vi "LinkamStageController.vi"() -> ()   [LabVIEW 2013]
doc: "The Grab and Save to AVI VI acquires images continuously using the high-level acquisition VIs, displays them in an image control, and saves the images to an AVI file. A grab is appropriate for high-speed applications that process only one image at a time. Use an AVI file to save multiple images to a single file for post-processing or record images.\n\nIMAQ Init initializes the device. IMAQ Grab Setup initializes the grab function and starts capturing images to an internal software buffer. IMAQ Create creates an image buffer IMAQ Grab Acquire copies the internal buffer to Image out, and an image control displays the image on the front panel. IMAQ Close releases resources associated with the acquisition, and IMAQ Dispose frees the image buffer.\n\nIMAQ AVI Create initializes the AVI file, IMAQ AVI WriteFrame adds each image to the AVI file, and IMAQ AVI Close completes writing to the AVI file. Call IMAQ AVI Create for each AVI file created."
uses:
  <vilib>/userdefined/High Color/IMAQdx.ctl
  Mag.ctl
  <vilib>/Instr/_visa.llb/VISA Open Access Mode.ctl
  ImageEnum4GFV.ctl
  RampProgramModel/RampProgramModel.lvclass
  AVI recoder state.ctl
  <vilib>/vision/Avi.llb/IMAQ AVI2 Refnum.ctl
  DateandTime.ctl
  RampProgramModel/RampProgramModel.lvclass/RampProgramModel.ctl
  TextOnImage.ctl
  Ascii Experiment Data.ctl
  RampState.ctl
  <vilib>/Instr/_visa.llb/VISA Configure Serial Port (Instr).vi
  <vilib>/Utility/file.llb/Read From Spreadsheet File (DBL).vi
  <vilib>/Utility/file.llb/Write To Spreadsheet File (string).vi
  <vilib>/vision/driver/NI_Vision_Acquisition_Software.lvlib
  <resource>/objmgr/imaqdx.rc
panel:
  in  "Stop Recording\n@ Temp (°C)":dbl=5.0 format="%#_g °C"
  in  "Start Recording\n@ Temp (°C)":dbl=-2.0 format="%#_g °C"
  in  "Enable\nAutomatic\nRecording":bool=TRUE
  in  "Gain (0-570)":dbl=300.0 min=0.0 max=570.0 step=1.0
  in  "Shutter (1-4095)":dbl=4095.0 min=1.0 max=4095.0 step=1.0
  in  "High Resolution":bool
  in  "Remarks":string
  out "Goal":string
  out "Experiment Name":string
  in  "NewExperiment":bool
  out "File Path":path=path "E:/LINKAM Measurements_Naama"
  in  "Mag":T1=enum."20x_LM"
  out "Temp Chart":dbl(graph)
  out "Time Remaining\n(HH:MM:SS)":dbl format="%<%H:%M:%S>t"
  out "Ramp Program Table":string[][](table)
  in  "Clear Table":bool
  in  "Add Entry":bool
  in  "StopProgram":bool
  in  "RunProgram":bool
  in  "PauseProgram":bool
  in  "SaveProgram":bool
  in  "LoadProgram":bool
  in  "Cycles":u32=1 min=1 max=1000 step=1
  out "Cycle No.":u32 min=1 max=1000 step=1
  in  "Pump Speed":u8(slide) max=30 step=1 scale=0.0..30.0
  in  "DelayInComm(ms)":u32=50
  out "Video Grabber":bool
  out "Linkam Controller":bool
  out "Ramp Controller":bool
  out "Video Recorder":bool
  in  "Pause":bool caption="Start Cooling/Heating"
  in  "Stop":bool caption="Start Cooling/Heating"
  in  "Record":bool caption="Start Cooling/Heating"
  out "Status":string="Stop"
  in  "TakeRefImage":bool caption="Start Cooling/Heating"
  in  "Time Between Consecutive Frames (sec)":dbl=1.0 caption="Time Between \nConsecutive \nFrames (sec)" min=0.0 max=3600.0 step=0.01 format="%.2g s"
  out "Full avi Path and Name":path=path "Z:/Downloads/data/Test-18_05_2014-15_02_54.avi"
  out "Codec Type":string="Motion JPEG (NI Vision)"
  in  "index 2":i32=4
  in  "error in (no error) 2":errorcluster
  out "Status":string="Stopped"
  out "Repeat Program ind":u32=1 min=1 max=1000 step=1
  in  "error in (no error)":errorcluster
  out "Reference Image":T2(plugin-control)
  in  "Hold Cooling/Heating":bool caption="Start Cooling/Heating"
  in  "Stop Cooling/Heating":bool caption="Start Cooling/Heating"
  in  "Start Cooling/Heating":bool
  in  "Setpoint (°C)":dbl=28.0 min=-50.0 max=50.0 step=0.1 format="%.1g °C"
  in  "Cooling Rate (°C/min)":dbl=1.0 min=0.0 max=20.0 step=0.01 format="%.2g °C/min"
  out "Current Temp (°C)":dbl=27.0 format="%.1g °C"
  out "Status of Liquied Nitrogen Pump":string="33"
  in  "Max Speed":bool
  in  "LNP mode":bool=TRUE
  out "Error Message":string
  out "Status of Temperature Controller":string="Setpoint"
  out "Temp String (C)":string="27.0"
  out "Timer":u32=9
  out "remaining string":string="010E"
  out "read buffer":string="0€Á€€€010E\r"
  out "return count":u32=11
  in  "Session In":T3="cam0"
  out "Image":T2(plugin-control)
  in  "stop":bool
  # "Live Image"
  # "Reference Image"
  # "Select your Camera above"
  # "Linkam Temperature Controller"
  # "Experiment Data"
  # "Video Recorder"
  # "Engines Status"
  # "Status"
  # "Liquid Nitrogen Pump Controller"
  # "Pump Speed"
  # "Video Grabber"
  # "Error Message"
  # "Ramp Table Controller"
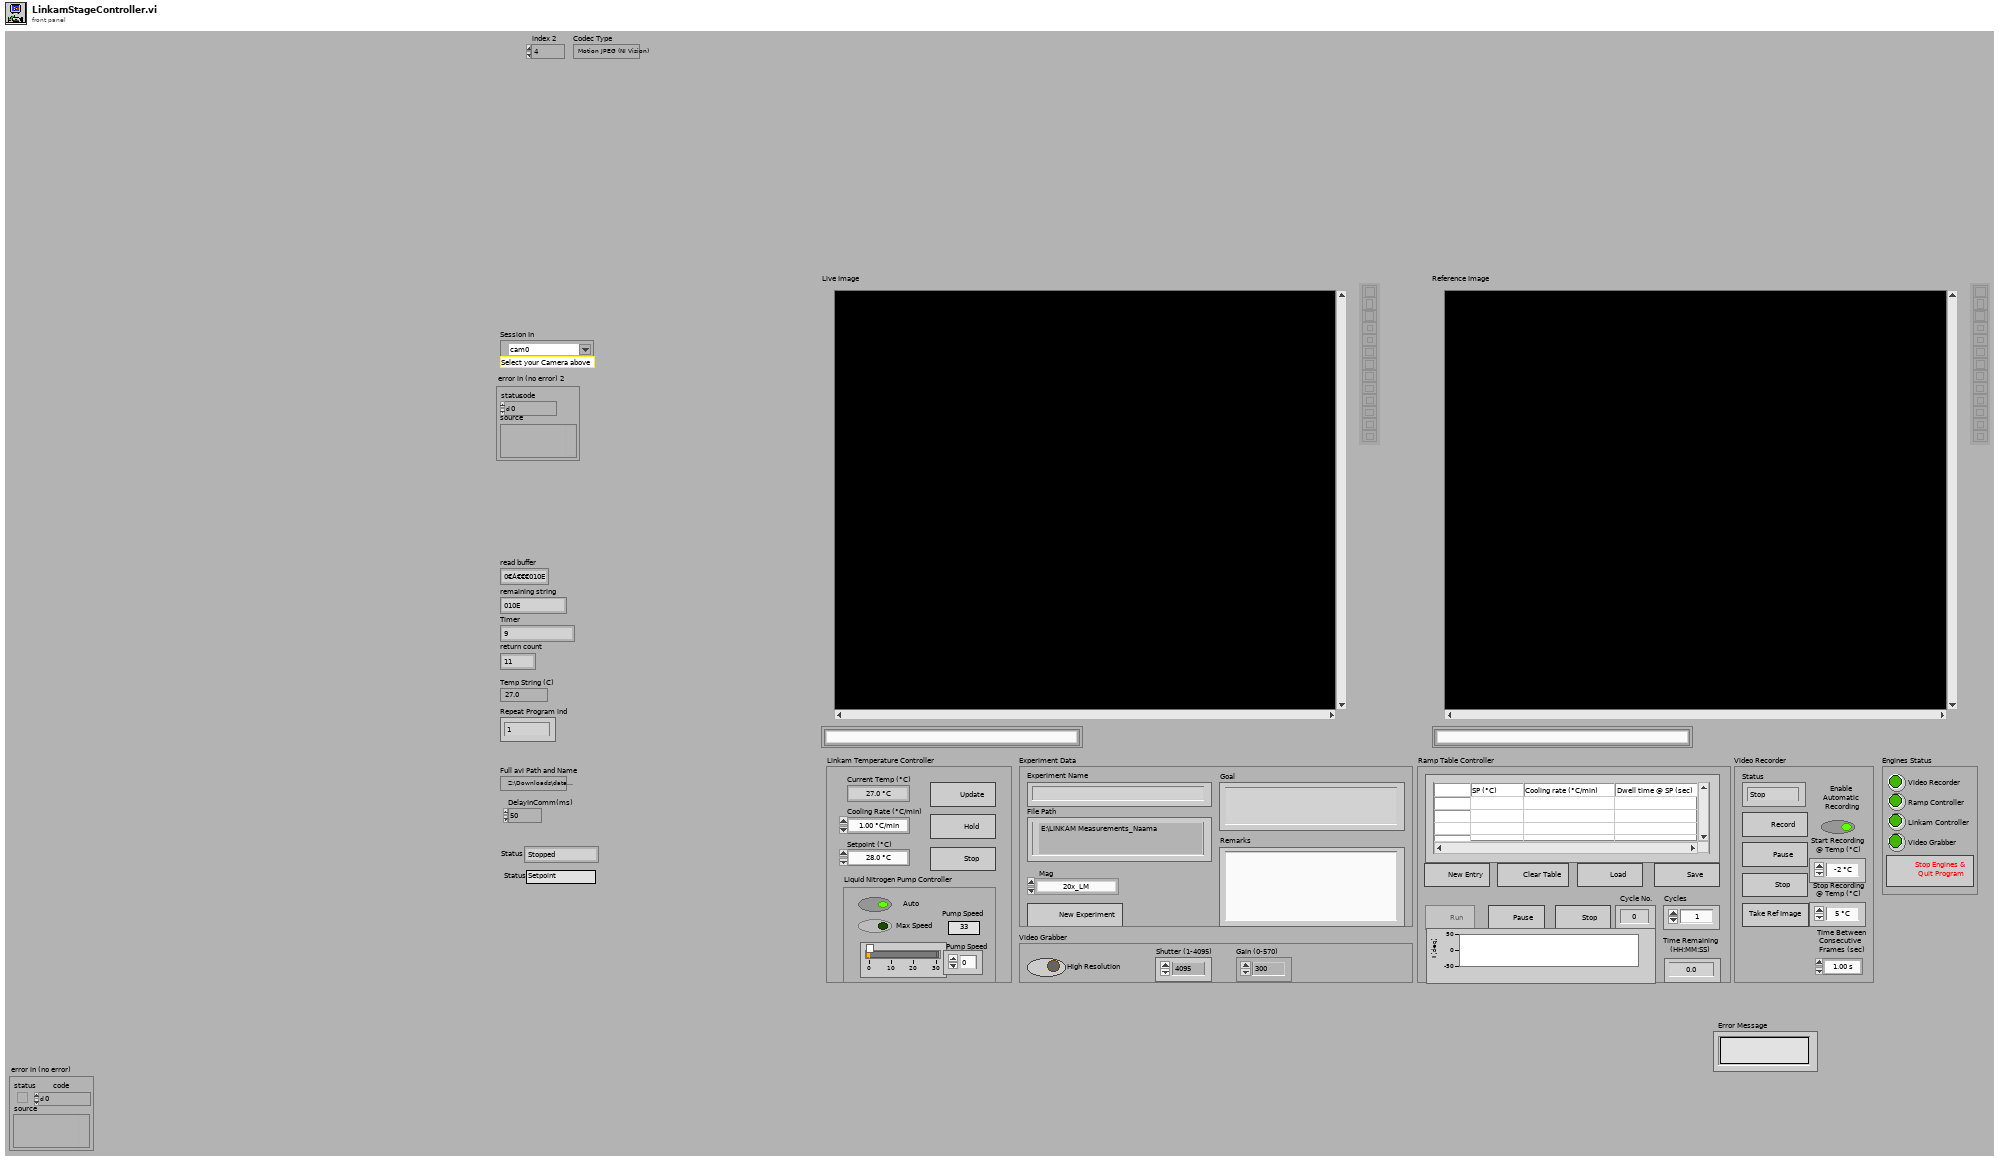
[diagram p1: front panel]
types:
  T1 = typedef "Mag.ctl" = enum16{"5x_M_BD", "10x_M", "10xM_BD", "10x_ph1", "20x_S", "20x_LM", "50x_S"}
  T2 = typedef "IMAQ Image.ctl" = refnum<image>
  T3 = typedef "IMAQdx.ctl" = refnum<k21>
  T4 = enum8{"Enabled", "Disabled", "Disabled and Grayed Out"}
  T5 = typedef "DateandTime.ctl" = cluster{"Date and Time":string, "Temp (deg)":string}[]
  T6 = typedef "IMAQ AVI2 Refnum.ctl" = refnum<k20>
  T7 = typedef "AVI recoder state.ctl" = enum16{"Record", "Pause", "Stop", "Init"}
  T8 = typedef "ImageEnum4GFV.ctl" = enum16{"Delete", "Write", "Read", "Init"}
  T9 = typedef "VISA Open Access Mode.ctl" = u32
  T10 = typedef "RampState.ctl" = enum16{"Pause Program", "Heatling/Cooling", "Dwelling @ SP", "Stopped"}
  T11 = typedef "Ascii Experiment Data.ctl" = cluster{"Experiment Name":string, "Goal":string, "Remarks":string, "File Path":string, "Mag":string, "Repeat Program Number":string, "Full avi Path and Name":path, "Ramp Table ":string[][], "Date and Time":T5}
  T12 = cluster{"date/time string":string, "Temp String (C)":string}
  T13 = typedef "TextOnImage.ctl" = cluster{"Status":string, "Experiment Name":string, "Current Temp (C)":string, "Set Point (C)":string, "Cooling Rate (C/min)":string, "Mag":T1}
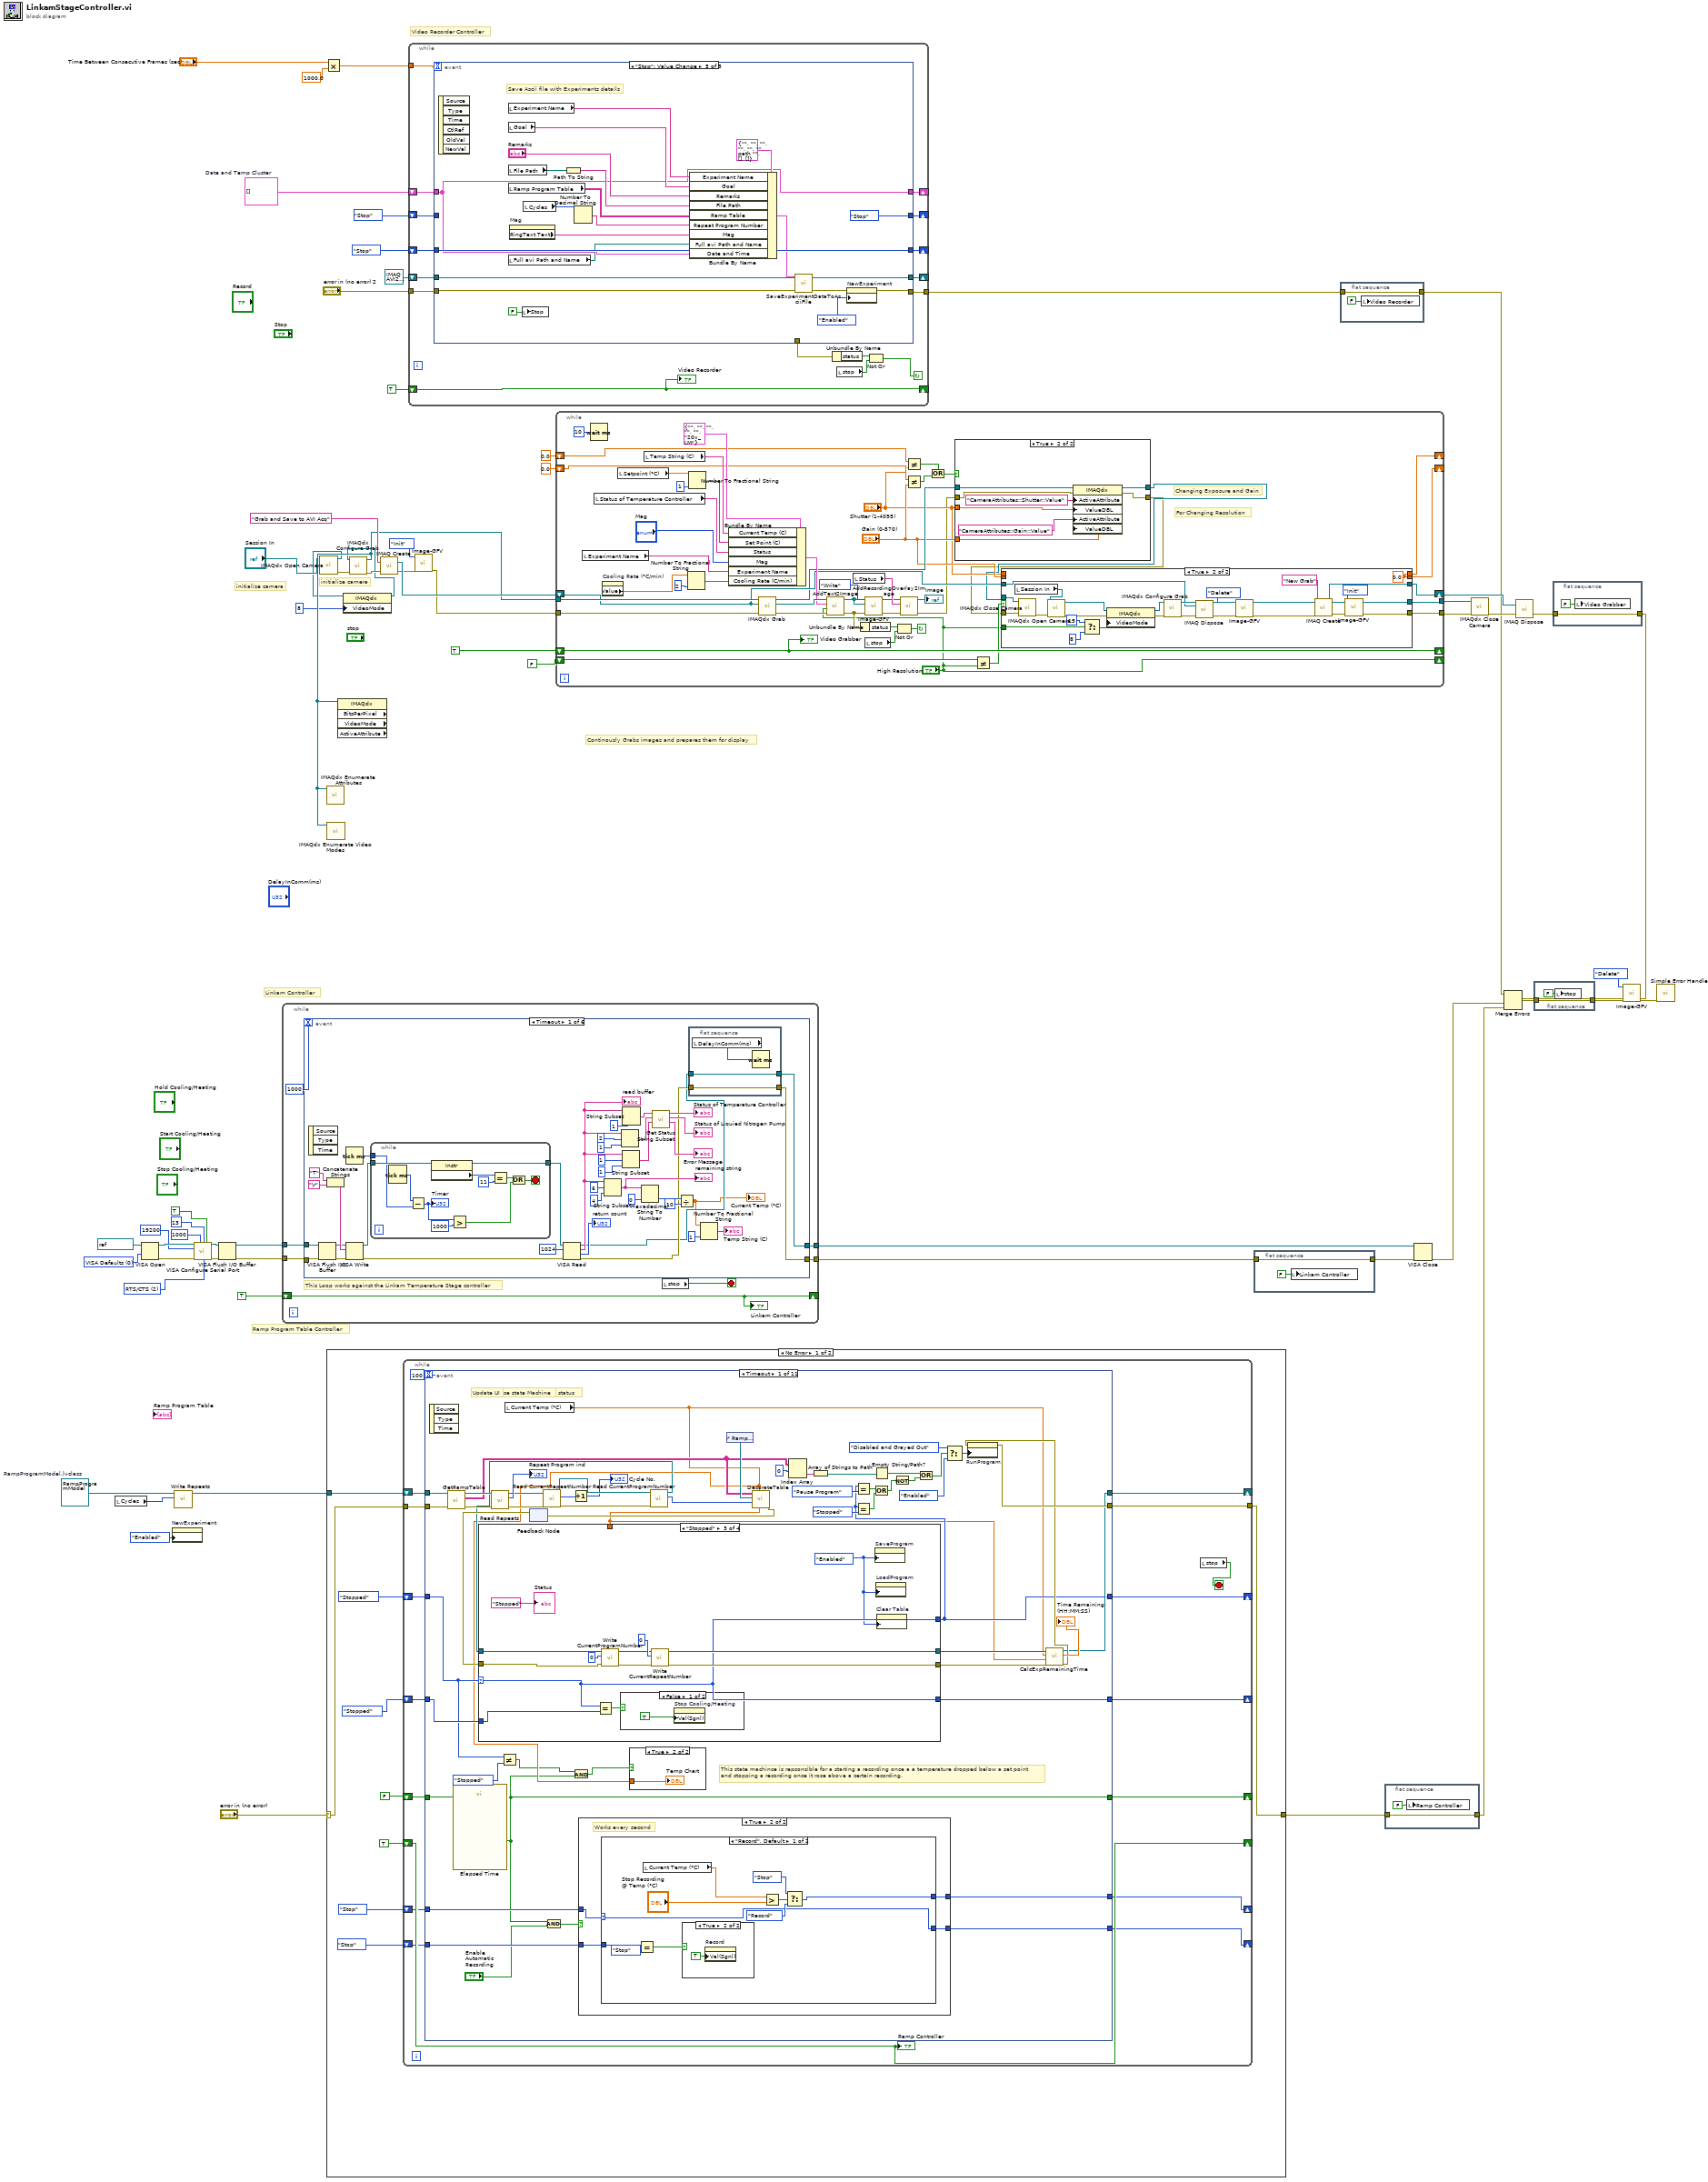
[diagram p0: block diagram]
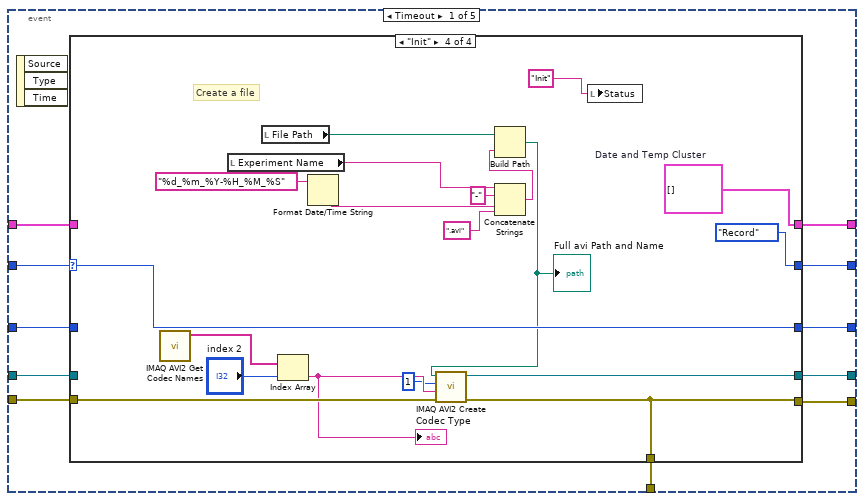
[diagram p2: hidden frame]
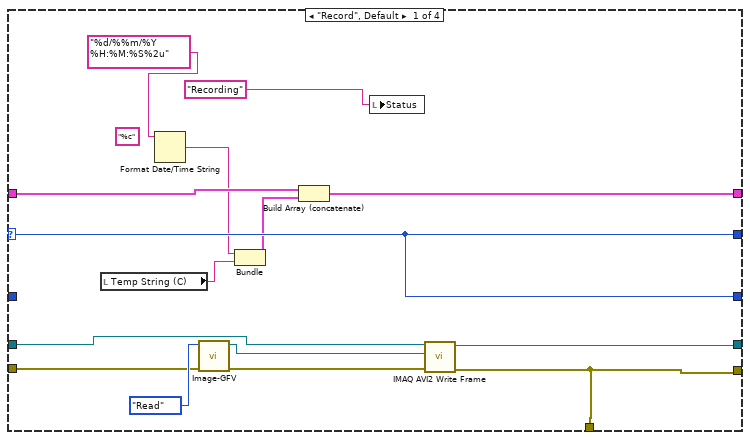
[diagram p3: hidden frame]
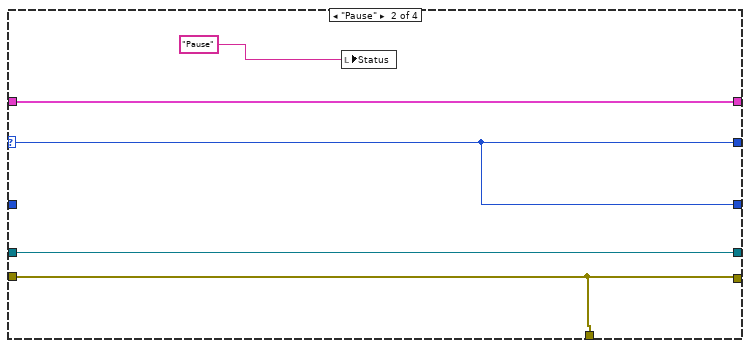
[diagram p4: hidden frame]
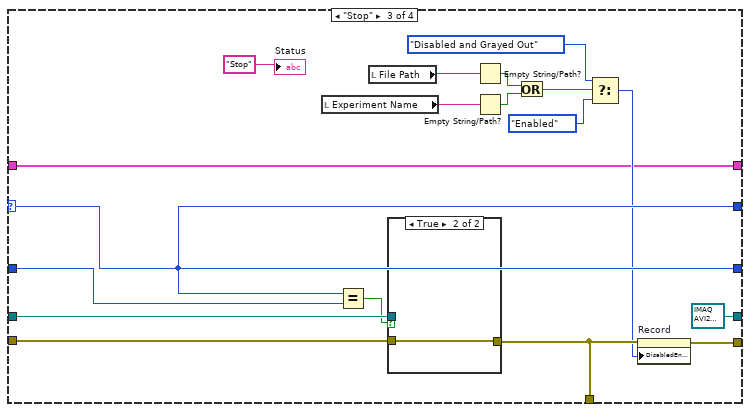
[diagram p5: hidden frame]
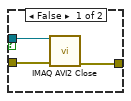
[diagram p6: hidden frame]
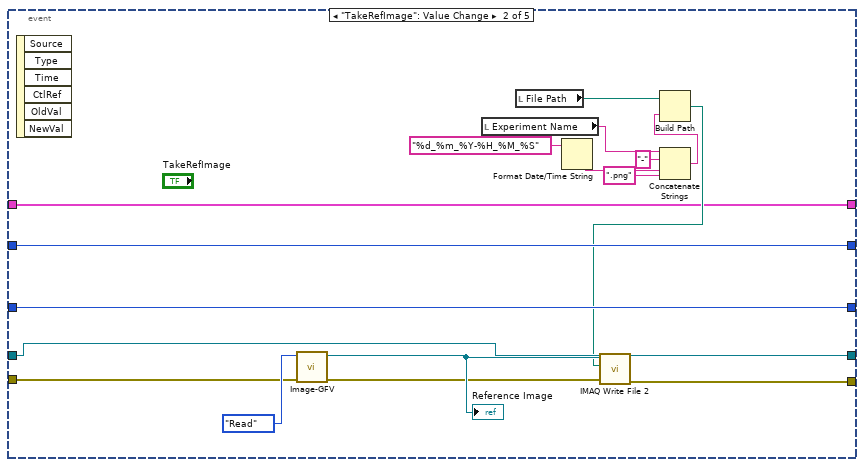
[diagram p7: hidden frame]
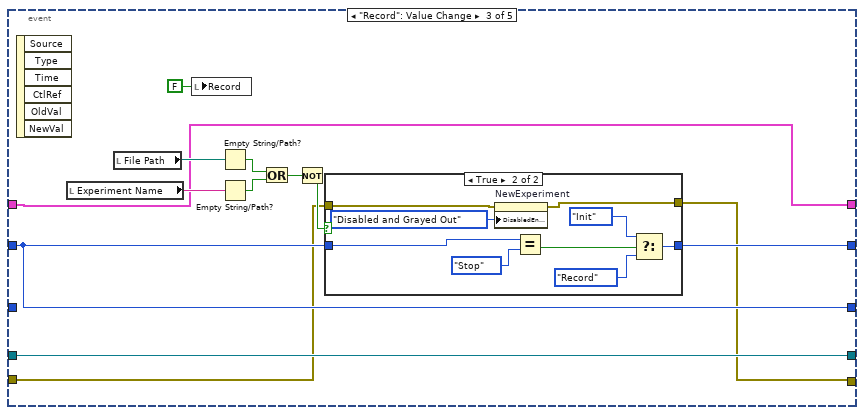
[diagram p8: hidden frame]
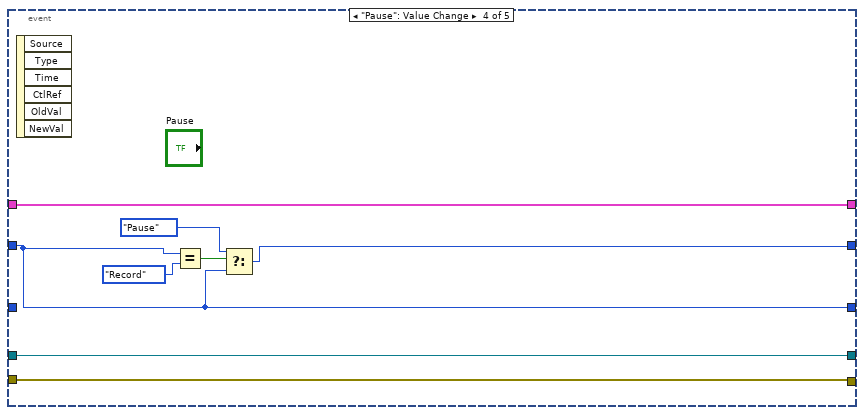
[diagram p10: hidden frame]
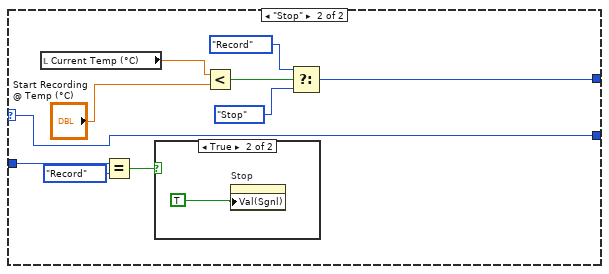
[diagram p13: hidden frame]
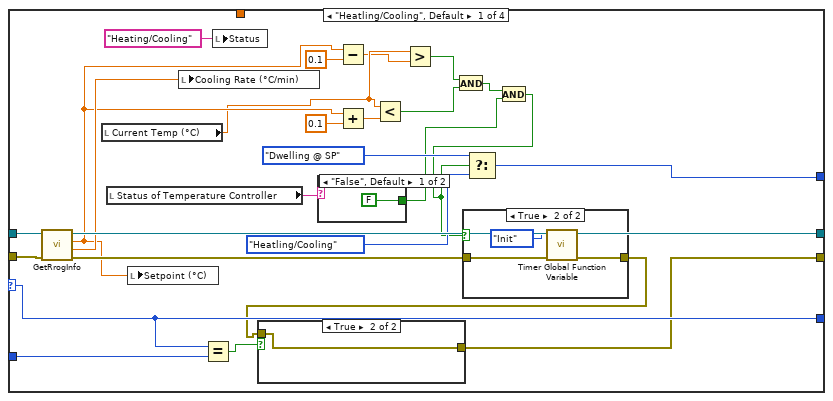
[diagram p16: hidden frame]
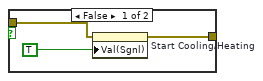
[diagram p17: hidden frame]
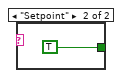
[diagram p18: hidden frame]
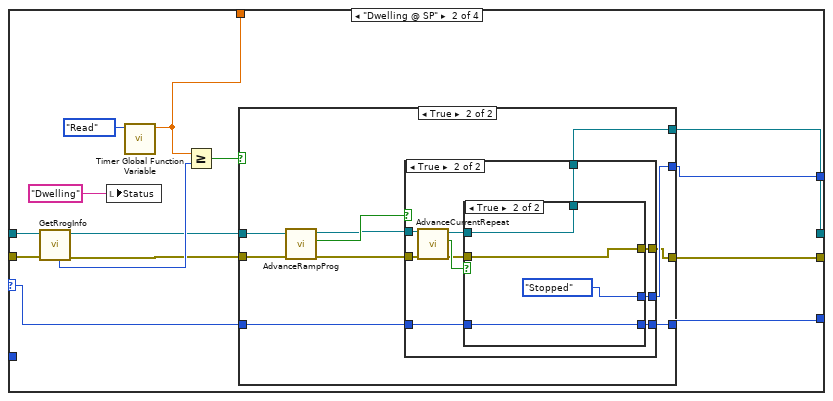
[diagram p20: hidden frame]
diagram:
  w11 = T5 []  # Date and Temp Cluster
  w33 = refnum<class "RampProgramModel.lvclass"> refnum  # RampProgramModel.lvclass
  w53 = T9 0 items=["VISA Defaults"=0, "Exclusive Lock"=1, "Load Configured Settings"=4] ("Access Mode")
  w57 = u16 2 items=["None", "XON/XOFF", "RTS/CTS", "XON/XOFF & RTS/CTS", "DTR/DSR", "XON/XOFF & DTR/DSR"] ("flow control (0:none)")
  # "Linkam Controller"
  # "Video Recorder Controller"
  # "Ramp Program Table Controller"
  # "Continously Grabs images and prepares them for display"
  # "initialize camera"
  # "initialize camera"
  n1 = local read "Cycles"() -> (w34:u32)
  n2 = VISA Open(access mode=w53, VISA resource name=refnum<visa-resource-name> "COM1") -> (VISA resource name=w60:refnum<visa-resource-name>, error out=w61:errorcluster)  [unwired: 3 in]
  n3 = property on="NewExperiment" class="Bool"("DisabledEnum"=T4."Enabled" ("Disabled")) -> ()  [unwired: 2 in, 2 out]
  n4 = call "Write Repeats.vi"("Repeats"=w34, "RampProgramModel in"=w33) -> ("RampProgramModel out"=w32:refnum<class "RampProgramModel.lvclass">)  [unwired: 8 in, 1 out]
  n5 = call-poly "VISA Configure Serial Port"("VISA resource name"=w60, "timeout (10sec)"=u32 1000, "termination char\n(0xA = '\\n' = LF)"=u8 13 ("termination char\n(0xA = '\\n' = LF)"), "Enable Termination\nChar (T)"=TRUE ("Enable Termination\nChar (T)"), "baud rate (9600)"=u32 19200, "error in (no error)"=w61, "flow control (0:none)"=w57) -> ("VISA resource name out"=w52:refnum<visa-resource-name>, "error out"=w51:errorcluster)  [unwired: 7 in]
  n6 = VISA Flush I/O Buffer(VISA resource name=w52, error in (no error)=w51) -> (VISA resource name out=w50:refnum<visa-resource-name>, error out=w49:errorcluster)  [unwired: 1 in]
  n7 = while {
    tunnel: [w69] -> w55
    tunnel: [w68] -> w17
    tunnel: w50 -> [w67]
    tunnel: w49 -> [w66]
    shift-right: [w63] -> _
    shift-left: TRUE -> [w63]
    stop <- w65 stop-if-true
    # "This Loop works against the Linkam Temperature Stage controller"
    n8 = event shown="[0] Timeout" {
      selector: _ -> [_ _ _ _ _ _]
      dyn-events: _ -> [_ _ _ _ _ _]
      timeout: 1000 -> [_ _ _ _ _ _]
      tunnel: [w72 w123 w136 w160 w182 w186] -> w69
      tunnel: [w71 w122 w135 w159 w183 w185] -> w68
      tunnel: w67 -> [w92 w131 w144 w171 w182 w210]
      tunnel: w66 -> [w91 w130 w143 w170 w183 w209]
      event Timeout {
        n9 = event-data() -> ()  [unwired: 1 in, 3 out]
        n10 = VISA Flush I/O Buffer(VISA resource name=w92, error in (no error)=w91) -> (VISA resource name out=w90:refnum<visa-resource-name>, error out=w89:errorcluster)  [unwired: 1 in]
        n11 = Concatenate Strings("T" ("write buffer"), "\r") -> (w93:string)
        n12 = Tick Count (ms)() -> (millisecond timer value=w96:u32)
        n13 = VISA Write(VISA resource name=w90, write buffer=w93, error in (no error)=w89) -> (VISA resource name out=w99:refnum<visa-resource-name>, error out=w97:errorcluster)  [unwired: 1 out]
        n14 = while {
          tunnel: w99 -> [w114]
          tunnel: [w113] -> w98
          tunnel: w96 -> [w112]
          stop <- w115 stop-if-true
          n15 = Tick Count (ms)() -> (millisecond timer value=w119:u32)
          n16 = Subtract(x=w119, y=w112) -> (x-y=w111:u32)
          "Timer" <- w111
          n17 = property class="Instr"(reference=w114) -> (reference out=w113:refnum<visa-resource-name>, "Serial Settings:Number of Bytes at Serial Port"=w121:u32)  [unwired: 1 in, 1 out]
          n18 = Greater?(x=w111, y=u32 1000) -> (0:w116:bool)
          n19 = Equal?(x=w121, y=u32 11) -> (x = y?=w117:bool)
          n20 = Or(x=w117, y=w116) -> (x .or. y?=w115:bool)
        }
        n21 = VISA Read(VISA resource name=w98, byte count=u32 1024, error in (no error)=w97) -> (VISA resource name out=w73:refnum<visa-resource-name>, read buffer=w77:string, return count=→"return count":u32, error out=w74:errorcluster)
        "read buffer" <- w77
        n22 = String Subset(string=w77, offset (0)=6, length (rest)=4 ("length (rest)")) -> (substring=w102:string)
        "remaining string" <- w102
        n23 = String Subset(string=w77, offset (0)=2, length (rest)=1 ("length (rest)")) -> (substring=w81:string)
        n24 = String Subset(string=w77, offset (0)=1, length (rest)=1 ("length (rest)")) -> (substring=w76:string)
        n25 = String Subset(string=w77, length (rest)=1 ("length (rest)")) -> (substring=w85:string)  [unwired: 1 in]
        n26 = Hexadecimal String To Number(string=w102, default (0uL)=i16 0 ("default (0 U32)")) -> (number=w101:i16)  [unwired: 1 in, 1 out]
        n27 = call "Get Status.vi"("Error message input"=w76, "Input Pump Status string"=w81, "Input Status String"=w85) -> ("Error message string"=→"Error Message":string, "Output Pump Status"=→"Status of Liquied Nitrogen Pump":string, "Output Status String"=→"Status of Temperature Controller":string)  [unwired: 6 in]
        n28 = Divide(x=w101, y=i16 10) -> (x/y=w70:dbl)
        "Current Temp (°C)" <- w70
        n29 = flat-sequence {
          tunnel: w74 -> [w110]
          tunnel: [w110] -> w71
          tunnel: w73 -> [w109]
          tunnel: [w109] -> w72
          frame #0 {
            n30 = local read "DelayInComm(ms)"() -> (w108:u32)
            n31 = Wait (ms)(milliseconds to wait=w108) -> ()  [unwired: 1 out]
          }
        }
        n32 = Number To Fractional String(number=w70, precision (6)=i16 1) -> (F-format string=→"Temp String (C)":string)  [unwired: 2 in]
      }
      event "Stop Cooling/Heating": Value Change {
        n33 = event-data() -> ()  [unwired: 1 in, 6 out]
        n34 = Concatenate Strings("E" ("write buffer"), "\r") -> (w127:string)
        n35 = VISA Write(VISA resource name=w131, write buffer=w127, error in (no error)=w130) -> (VISA resource name out=w125:refnum<visa-resource-name>, error out=w124:errorcluster)  [unwired: 1 out]
        n36 = flat-sequence {
          tunnel: w124 -> [w134]
          tunnel: [w134] -> w122
          tunnel: w125 -> [w133]
          tunnel: [w133] -> w123
          frame #0 {
            n37 = local read "DelayInComm(ms)"() -> (w132:u32)
            n38 = Wait (ms)(milliseconds to wait=w132) -> ()  [unwired: 1 out]
          }
        }
        n39 = local write "Stop Cooling/Heating"(FALSE ("Stop Cooling/Heating")) -> ()
      }
      event "Hold Cooling/Heating": Value Change {
        n40 = event-data() -> ()  [unwired: 1 in, 6 out]
        n41 = Concatenate Strings("OCR" ("write buffer"), "\r") -> (w140:string)
        n42 = VISA Write(VISA resource name=w144, write buffer=w140, error in (no error)=w143) -> (VISA resource name out=w138:refnum<visa-resource-name>, error out=w137:errorcluster)  [unwired: 1 out]
        n43 = local write "Hold Cooling/Heating"(FALSE ("Hold Cooling/Heating")) -> ()
        n44 = flat-sequence {
          tunnel: w137 -> [w147]
          tunnel: [w147] -> w135
          tunnel: w138 -> [w146]
          tunnel: [w146] -> w136
          frame #0 {
            n45 = local read "DelayInComm(ms)"() -> (w145:u32)
            n46 = Wait (ms)(milliseconds to wait=w145) -> ()  [unwired: 1 out]
          }
        }
      }
      event "LNP mode", "Pump Speed": Value Change {
        n47 = event-data() -> ()  [unwired: 1 in, 6 out]
        n48 = Select(t="Pa0", s="LNP mode", f="Pm0") -> (s? t:f=w166:string)
        n49 = Concatenate Strings(w166, "\r") -> (w168:string)
        n50 = VISA Write(VISA resource name=w171, write buffer=w168, error in (no error)=w170) -> (VISA resource name out=w158:refnum<visa-resource-name>, error out=w157:errorcluster)  [unwired: 1 out]
        n51 = flat-sequence {
          tunnel: w157 -> [w174]
          tunnel: [w174] -> w156
          tunnel: w158 -> [w173]
          tunnel: [w173] -> w155
          frame #0 {
            n52 = local read "DelayInComm(ms)"() -> (w172:u32)
            n53 = Wait (ms)(milliseconds to wait=w172) -> ()  [unwired: 1 out]
          }
        }
        n54 = Add(x="Pump Speed", y=u8 48) -> (x+y=w152:u8)
        n55 = Type Cast(x=w152) -> (*(type *) &x=w150:string)  [unwired: 1 out]
        n56 = Concatenate Strings("P" ("string"), w150) -> (w149:string)
        n57 = Concatenate Strings(w149, "\r") -> (w163:string)
        n58 = VISA Write(VISA resource name=w155, write buffer=w163, error in (no error)=w156) -> (VISA resource name out=w162:refnum<visa-resource-name>, error out=w161:errorcluster)  [unwired: 1 out]
        n59 = flat-sequence {
          tunnel: w161 -> [w177]
          tunnel: [w177] -> w159
          tunnel: w162 -> [w176]
          tunnel: [w176] -> w160
          frame #0 {
            n60 = local read "DelayInComm(ms)"() -> (w175:u32)
            n61 = Wait (ms)(milliseconds to wait=w175) -> ()  [unwired: 1 out]
          }
        }
      }
      event "Max Speed": Value Change {
        n62 = event-data() -> ()  [unwired: 1 in, 6 out]
        n63 = Select(t=u8 30 ("f"), s="Max Speed", f=u8 0) -> (s? t:f=w180:u8)
        n64 = property on="Pump Speed" class="Slide (strict)"("Val(Sgnl)"=w180) -> ()  [unwired: 2 in, 2 out]
      }
      event "Start Cooling/Heating": Value Change {
        # "Caused to max speed at every update"
        n65 = event-data() -> ()  [unwired: 1 in, 6 out]
        n66 = Multiply(x="Cooling Rate (°C/min)", y=u16 100) -> (x*y=w199:dbl)
        n67 = To Long Integer(number=w199) -> (32bit integer=w198:i32)
        n68 = Number To Decimal String(number=w198) -> (decimal integer string=w211:string)  [unwired: 1 in]
        n69 = property on="LNP mode" class="Bool (strict)"() -> ("Value"=w184:bool)  [unwired: 2 in, 2 out]
        n70 = Concatenate Strings("R1" ("write buffer"), w211, "\r") -> (w208:string)
        n71 = VISA Write(VISA resource name=w210, write buffer=w208, error in (no error)=w209) -> (VISA resource name out=w195:refnum<visa-resource-name>, error out=w196:errorcluster)  [unwired: 1 out]
        n72 = case shown="False" w184 {
          frame False {
            n73 = property on="LNP mode" class="Bool (strict)"("Val(Sgnl)"=TRUE ("LNP mode")) -> ()  [unwired: 2 in, 2 out]
          }
          frame True {
          }
        }
        n74 = flat-sequence {
          tunnel: w196 -> [w227]
          tunnel: [w227] -> w193
          tunnel: w195 -> [w226]
          tunnel: [w226] -> w194
          frame #0 {
            n75 = local read "DelayInComm(ms)"() -> (w225:u32)
            n76 = Wait (ms)(milliseconds to wait=w225) -> ()  [unwired: 1 out]
          }
        }
        n77 = local write "Start Cooling/Heating"(FALSE ("Start Cooling/Heating")) -> ()
        n78 = Multiply(x="Setpoint (°C)", y=u16 10) -> (x*y=w206:dbl)
        n79 = Number To Decimal String(number=w206) -> (decimal integer string=w207:string)  [unwired: 1 in]
        n80 = Concatenate Strings("L1" ("write buffer"), w207, "\r") -> (w201:string)
        n81 = VISA Write(VISA resource name=w194, write buffer=w201, error in (no error)=w193) -> (VISA resource name out=w192:refnum<visa-resource-name>, error out=w191:errorcluster)  [unwired: 1 out]
        n82 = flat-sequence {
          tunnel: w191 -> [w224]
          tunnel: [w224] -> w189
          tunnel: w192 -> [w223]
          tunnel: [w223] -> w190
          frame #0 {
            n83 = local read "DelayInComm(ms)"() -> (w222:u32)
            n84 = Wait (ms)(milliseconds to wait=w222) -> ()  [unwired: 1 out]
          }
        }
        n85 = flat-sequence {
          tunnel: w187 -> [w221]
          tunnel: [w221] -> w185
          tunnel: w188 -> [w220]
          tunnel: [w220] -> w186
          frame #0 {
            n86 = local read "DelayInComm(ms)"() -> (w219:u32)
            n87 = Wait (ms)(milliseconds to wait=w219) -> ()  [unwired: 1 out]
          }
        }
        n88 = Concatenate Strings("S" ("write buffer"), "\r") -> (w215:string)
        n89 = VISA Write(VISA resource name=w190, write buffer=w215, error in (no error)=w189) -> (VISA resource name out=w188:refnum<visa-resource-name>, error out=w187:errorcluster)  [unwired: 1 out]
      }
    }
    n90 = local read "stop"() -> (w65:bool)
    "Linkam Controller" <- w63
  }
  n91 = call <vilib>:"IMAQdx Open Camera.vi"("Session In"="Session In") -> ("error out"=w47:errorcluster, "Session Out"=w7:T3)  [unwired: 2 in, 7 out]
  n92 = Multiply(x="Time Between Consecutive Frames (sec)", y=1000.0) -> (x*y=w29:dbl)
  n93 = case shown="No Error" "error in (no error)" {
    selector: "error in (no error)" -> [w236 w545]
    tunnel: [w235 w545] -> w19
    tunnel: w32 -> [w234 _]
    frame No Error {
      n94 = while {
        tunnel: w236 -> [w253]
        tunnel: [w252] -> w235
        shift-right: [w250] -> _
        shift-left: w234 -> [w251]
        shift-right: [w247] -> _
        shift-left: RampState."Stopped" ("State") -> [w248]
        shift-right: [w245] -> _
        shift-left: RampState."Stopped" ("State") -> [w244]
        shift-right: [w243] -> _
        shift-left: TRUE -> [w243]
        shift-right: [w241] -> _
        shift-left: FALSE -> [w242]
        shift-right: [w238] -> _
        shift-left: AVI_recoder_state."Stop" -> [w240]
        shift-right: [w237] -> _
        shift-left: AVI_recoder_state."Stop" -> [w239]
        stop <- w246 stop-if-true
        n95 = event shown="[0] Timeout" {
          selector: _ -> [_ _ _ _ _ _ _ _ _ _ _]
          dyn-events: _ -> [_ _ _ _ _ _ _ _ _ _ _]
          timeout: u32 100 ("milliseconds to wait") -> [_ _ _ _ _ _ _ _ _ _ _]
          tunnel: w253 -> [w307 w454 w466 w475 w483 w490 w496 w505 w512 w525 w542]
          tunnel: [w290 w453 w466 w474 w483 w488 w496 w505 w512 w520 w541] -> w252
          tunnel: w251 -> [w306 w457 w467 w476 w482 w491 w497 w506 w511 w518 w543]
          tunnel: [w280 w457 w467 w473 w481 w489 w497 w506 w511 w519 w540] -> w250
          tunnel: w248 -> [w267 w456 w465 w471 w479 w486 _ _ _ w517 w544]
          tunnel: [w275 w456 w465 w471 w479 w486 RampState."Pause Program" ("State") RampState."Heatling/Cooling" ("State") RampState."Stopped" ("State") w517 w544] -> w247
          tunnel: [w298 w455 w464 w471 w479 w486 w494 w502 w510 w516 w538] -> w245
          tunnel: w244 -> [w297 w455 w464 _ _ _ w494 w502 w510 w516 w538]
          tunnel: w242 -> [w263 _ _ _ _ _ _ _ _ _ _]
          tunnel: [w254 _ _ _ _ _ _ _ _ _ _] -> w241
          tunnel: w240 -> [w260 w448 w463 w470 w478 w485 w493 w499 w509 w515 w537]
          tunnel: w239 -> [w259 w447 w462 w469 w477 w484 w492 w498 w508 w514 w536]
          tunnel: [w258 w448 w463 w470 w478 w485 w493 w499 w509 w515 w537] -> w238
          tunnel: [w255 w447 w462 w469 w477 w484 w492 w498 w508 w514 w536] -> w237
          event Timeout {
            # "This state machince is repsonsible for a starting a recording once a a temperature dropped below a set point \nand stopping a recording once it rose above a certain recording."
            # "Read Current Temperture and status"
            # "And advance state Machine"
            # "Update UI"
            n96 = event-data() -> ()  [unwired: 1 in, 3 out]
            n97 = call "GetRampTable.vi"("error in (no error)"=w307, "RampProgramModel in"=w306) -> ("error out"=w303:errorcluster, "RampTable"=w296:string[][], "RampProgramModel out"=w305:refnum<class "RampProgramModel.lvclass">)  [unwired: 7 in]
            n98 = call "Elapsed Time"("Reset"=w263) -> ("Time has Elapsed"=w254:bool)  [unwired: 11 in, 7 out]
            n99 = call "Read Repeats.vi"("error in (no error)"=w303, "RampProgramModel in"=w305) -> ("error out"=w301:errorcluster, "Repeats"=→"Repeat Program ind":u32, "RampProgramModel out"=w302:refnum<class "RampProgramModel.lvclass">)  [unwired: 7 in]
            n100 = Not Equal?(x=w267, y=RampState."Stopped" ("State")) -> (x != y?=w261:bool)
            n101 = local read "Current Temp (°C)"() -> (w262:dbl)
            n102 = feedback #1() -> (w288:errorcluster)  [unwired: 1 in]
            n103 = call "Read CurrentRepeatNumber.vi"("error in (no error)"=w301, "RampProgramModel in"=w302) -> ("error out"=w285:errorcluster, "CurrentRepeatNumber"=w269:u32, "RampProgramModel out"=w286:refnum<class "RampProgramModel.lvclass">)  [unwired: 7 in]
            n104 = And(x=w254, y="Enable\nAutomatic\nRecording") -> (x .and. y?=w256:bool)
            n105 = Increment(x=w269) -> (x+1=→"Cycle No.":u32)
            n106 = And(x=w261, y=w254) -> (x .and. y?=w264:bool)
            n107 = case shown="True" w256 {
              tunnel: w260 -> [w309 w313]
              tunnel: w259 -> [w308 w312]
              tunnel: [w309 w311] -> w258
              tunnel: [w308 w310] -> w255
              frame False {
              }
              frame True {
                # "Works every second"
                n108 = case shown="\"Record\", Default" w313 {
                  selector: w313 -> [w315 w326]
                  tunnel: w312 -> [w323 w329]
                  tunnel: [w317 w331] -> w311
                  tunnel: [w315 w326] -> w310
                  frame "Record", Default {
                    n109 = Equal?(x=w323, y=AVI_recoder_state."Stop") -> (x = y?=w321:bool)
                    n110 = local read "Current Temp (°C)"() -> (w314:dbl)
                    n111 = case shown="True" w321 {
                      frame False {
                      }
                      frame True {
                        n112 = property on="Record" class="Bool (strict)"("Val(Sgnl)"=TRUE ("Value (Signaling)")) -> ()  [unwired: 2 in, 2 out]
                      }
                    }
                    n113 = Greater?(x=w314, y="Stop Recording\n@ Temp (°C)") -> (0:w320:bool)
                    n114 = Select(t=AVI_recoder_state."Stop" ("y"), s=w320, f=AVI_recoder_state."Record" ("y")) -> (s? t:f=w317:T7)
                  }
                  frame "Stop" {
                    n115 = local read "Current Temp (°C)"() -> (w325:dbl)
                    n116 = Equal?(x=w329, y=AVI_recoder_state."Record") -> (x = y?=w328:bool)
                    n117 = case shown="True" w328 {
                      frame False {
                      }
                      frame True {
                        n118 = property on="Stop" class="Bool (strict)"("Val(Sgnl)"=TRUE ("Value (Signaling)")) -> ()  [unwired: 2 in, 2 out]
                      }
                    }
                    n119 = Less?(x=w325, y="Start Recording\n@ Temp (°C)") -> (x < y?=w334:bool)
                    n120 = Select(t=AVI_recoder_state."Record", s=w334, f=AVI_recoder_state."Stop") -> (s? t:f=w331:T7)
                  }
                }
              }
            }
            n121 = case shown="True" w264 {
              tunnel: w262 -> [_ w336]
              frame False {
              }
              frame True {
                "Temp Chart" <- w336
              }
            }
            n122 = call "Read CurrentProgramNumber.vi"("error in (no error)"=w285, "RampProgramModel in"=w286) -> ("CurrentProgramNumber"=w299:u32, "RampProgramModel out"=w283:refnum<class "RampProgramModel.lvclass">)  [unwired: 7 in, 1 out]
            n123 = case shown="\"Stopped\"" w267 {
              selector: w267 -> [w352 w374 w430 w442]
              tunnel: [w357 w381 w430 w442] -> w275
              tunnel: w283 -> [w361 w385 w437 w444]
              tunnel: [w360 w378 w431 w444] -> w284
              tunnel: [w338 w377 w432 w440] -> w282
              tunnel: [_ w376 _ _] -> w265
              tunnel: [w352 w375 w430 w442] -> w298
              tunnel: w297 -> [w353 _ w429 w443]
              tunnel: w288 -> [w337 w373 w427 w440]
              frame "Heatling/Cooling", Default {
                n124 = call "GetRrogInfo.vi"("error in (no error)"=w337, "RampProgramModel in"=w361) -> ("error out"=w356:errorcluster, "Cooling rate (°C/min)"=w355:dbl, "SP (°C)"=w348:dbl, "RampProgramModel out"=w360:refnum<class "RampProgramModel.lvclass">)  [unwired: 5 in, 1 out]
                n125 = local read "Current Temp (°C)"() -> (w346:dbl)
                n126 = local read "Status of Temperature Controller"() -> (w354:string)
                n127 = local write "Setpoint (°C)"(w348) -> ()
                n128 = local write "Cooling Rate (°C/min)"(w355) -> ()
                n129 = Equal?(x=w352, y=w353) -> (x = y?=w351:bool)
                n130 = local write "Status"("Heating/Cooling" ("Status")) -> ()
                n131 = case shown="\"False\", Default" w354 {
                  tunnel: [FALSE TRUE] -> w341
                  frame "False", Default {
                  }
                  frame "Setpoint" {
                  }
                }
                n132 = Subtract(x=w348, y=0.1) -> (x-y=w345:dbl)
                n133 = Add(x=w348, y=0.1) -> (x+y=w347:dbl)
                n134 = Less?(x=w346, y=w347) -> (x < y?=w343:bool)
                n135 = Greater?(x=w346, y=w345) -> (0:w344:bool)
                n136 = And(x=w344, y=w343) -> (x .and. y?=w342:bool)
                n137 = And(x=w342, y=w341) -> (x .and. y?=w340:bool)
                n138 = case shown="True" w340 {
                  tunnel: w356 -> [w369 w371]
                  tunnel: [w369 w370] -> w339
                  frame False {
                  }
                  frame True {
                    n139 = call "Timer Global Function Variable.vi"("error in (no error)"=w371, "Enum"=enum16{"Init", "Read", "Set"}."Init") -> ("error out"=w370:errorcluster)  [unwired: 7 in, 2 out]
                  }
                }
                n140 = case shown="True" w351 {
                  tunnel: w339 -> [w364 w366]
                  tunnel: [w363 w366] -> w338
                  frame False {
                    n141 = property on="Start Cooling/Heating" class="Bool (strict)"(error in=w364, "Val(Sgnl)"=TRUE) -> (error out=w363:errorcluster)  [unwired: 1 in, 1 out]
                  }
                  frame True {
                  }
                }
                n142 = Select(t=RampState."Dwelling @ SP" ("State"), s=w340, f=RampState."Heatling/Cooling" ("State")) -> (s? t:f=w357:T10)
              }
              frame "Dwelling @ SP" {
                n143 = call "GetRrogInfo.vi"("error in (no error)"=w373, "RampProgramModel in"=w385) -> ("error out"=w379:errorcluster, "RampProgramModel out"=w380:refnum<class "RampProgramModel.lvclass">, "Dwell Time @ SP (sec)"=w383:u32)  [unwired: 5 in, 2 out]
                n144 = local write "Status"("Dwelling" ("Status")) -> ()
                n145 = call "Timer Global Function Variable.vi"("Enum"=enum16{"Init", "Read", "Set"}."Read") -> ("Time Elapsed"=w376:dbl)  [unwired: 8 in, 2 out]
                n146 = Greater Or Equal?(x=w376, y=w383) -> (x >= y?=w382:bool)
                n147 = case shown="True" w382 {
                  tunnel: [RampState."Dwelling @ SP" ("State") w395] -> w381
                  tunnel: w380 -> [w389 w400]
                  tunnel: w379 -> [w388 w399]
                  tunnel: [w389 w394] -> w378
                  tunnel: [w388 w393] -> w377
                  tunnel: [w387 w392] -> w375
                  tunnel: w374 -> [w387 w391]
                  frame False {
                  }
                  frame True {
                    n148 = call "AdvanceRampProg.vi"("error in (no error)"=w399, "RampProgramModel in"=w400) -> ("error out"=w396:errorcluster, "EndOfPrograms"=w398:bool, "RampProgramModel out"=w397:refnum<class "RampProgramModel.lvclass">)  [unwired: 7 in]
                    n149 = case shown="True" w398 {
                      tunnel: w397 -> [w402 w414]
                      tunnel: w396 -> [w403 w413]
                      tunnel: [RampState."Heatling/Cooling" ("State") w409] -> w395
                      tunnel: [w402 w408] -> w394
                      tunnel: [w403 w407] -> w393
                      tunnel: [w401 w406] -> w392
                      tunnel: w391 -> [w401 w405]
                      frame False {
                      }
                      frame True {
                        n150 = call "AdvanceCurrentRepeat.vi"("error in (no error)"=w413, "RampProgramModel in"=w414) -> ("error out"=w410:errorcluster, "EndOfRepeats"=w412:bool, "RampProgramModel out"=w411:refnum<class "RampProgramModel.lvclass">)  [unwired: 7 in]
                        n151 = case shown="True" w412 {
                          tunnel: w411 -> [w419 w423]
                          tunnel: w410 -> [w418 w424]
                          tunnel: [RampState."Heatling/Cooling" ("State") RampState."Stopped" ("State")] -> w409
                          tunnel: [w416 w423] -> w408
                          tunnel: [w417 w424] -> w407
                          tunnel: [w415 w422] -> w406
                          tunnel: w405 -> [w415 w422]
                          frame False {
                            n152 = call "Write CurrentProgramNumber.vi"("error in (no error)"=w418, "CurrentProgramNumber"=u32 0, "RampProgramModel in"=w419) -> ("error out"=w417:errorcluster, "RampProgramModel out"=w416:refnum<class "RampProgramModel.lvclass">)  [unwired: 7 in]
                          }
                          frame True {
                          }
                        }
                      }
                    }
                  }
                }
              }
              frame "Stopped" {
                w426 = T4."Enabled" ("Disabled")
                n153 = Equal?(x=w430, y=w429) -> (x = y?=w428:bool)
                n154 = call "Write CurrentProgramNumber.vi"("error in (no error)"=w427, "CurrentProgramNumber"=u32 0, "RampProgramModel in"=w437) -> ("error out"=w433:errorcluster, "RampProgramModel out"=w434:refnum<class "RampProgramModel.lvclass">)  [unwired: 7 in]
                n155 = case shown="False" w428 {
                  frame False {
                    n156 = property on="Stop Cooling/Heating" class="Bool (strict)"("Val(Sgnl)"=TRUE ("Value (Signaling)")) -> ()  [unwired: 2 in, 2 out]
                  }
                  frame True {
                  }
                }
                n157 = call "Write CurrentRepeatNumber.vi"("error in (no error)"=w433, "CurrentRepeatNumber"=u32 0, "RampProgramModel in"=w434) -> ("error out"=w432:errorcluster, "RampProgramModel out"=w431:refnum<class "RampProgramModel.lvclass">)  [unwired: 7 in]
                n158 = property on="SaveProgram" class="Bool"("DisabledEnum"=w426) -> ()  [unwired: 2 in, 2 out]
                n159 = property on="LoadProgram" class="Bool"("DisabledEnum"=w426) -> ()  [unwired: 2 in, 2 out]
                n160 = property on="Clear Table" class="Bool"("DisabledEnum"=w426) -> ()  [unwired: 2 in, 2 out]
                "Status" <- "Stopped" ("Status")
              }
              frame "Pause Program" {
                # "Send the hold command to the controller"
                n161 = Equal?(x=w442, y=w443) -> (x = y?=w441:bool)
                n162 = case shown="False" w441 {
                  frame False {
                    n163 = property on="Hold Cooling/Heating" class="Bool (strict)"("Val(Sgnl)"=TRUE ("Value (Signaling)")) -> ()  [unwired: 2 in, 2 out]
                  }
                  frame True {
                  }
                }
                n164 = local write "Status"("Pause" ("Status")) -> ()
              }
            }
            n165 = control-ref of="Ramp Program Table"() -> (w300:refnum<vi>)
            n166 = call "DecorateTable.vi"("Elapsed Time"=w265, "Current Temperature"=w262, "Current Program"=w299, "Tbl Refnum"=w300, "RampTable"=w296) -> ("error out"=w289:errorcluster)  [unwired: 6 in]
            n167 = feedback-in #1(w289) -> ()
            n168 = Index Array(array=w296, index (row)=0) -> (element=w294:string[])  [unwired: 1 in]
            n169 = Array of Strings to Path(0:w294) -> (2:w293:path)  [unwired: 1 in]
            n170 = Equal?(x=w275, y=RampState."Pause Program" ("State")) -> (x = y?=w274:bool)
            n171 = Equal?(x=w275, y=RampState."Stopped" ("State")) -> (x = y?=w277:bool)
            n172 = Empty String/Path?(string/path=w293) -> (empty?=w273:bool)
            n173 = Or(x=w274, y=w277) -> (x .or. y?=w271:bool)
            n174 = Not(x=w271) -> (.not. x?=w270:bool)
            n175 = Or(x=w273, y=w270) -> (x .or. y?=w272:bool)
            n176 = Select(t=T4."Disabled and Grayed Out" ("Disabled"), s=w272, f=T4."Enabled" ("Disabled")) -> (s? t:f=w291:T4)
            n177 = call "CalcExpRemainingTime.vi"("error in (no error)"=w282, "Current Dwell Time"=w265, "Current Temperature"=w262, "RampProgramModel in"=w284) -> ("error out"=w281:errorcluster, "RemainExpTime(sec)"=→"Time Remaining\n(HH:MM:SS)":dbl, "RampProgramModel out"=w280:refnum<class "RampProgramModel.lvclass">)  [unwired: 5 in]
            n178 = property on="RunProgram" class="Bool"(error in=w281, "DisabledEnum"=w291) -> (error out=w290:errorcluster)  [unwired: 1 in, 1 out]
          }
          event "NewExperiment": Value Change {
            n179 = event-data() -> ()  [unwired: 1 in, 6 out]
            n180 = call "NewExperimentDialog.vi"("error in (no error)"=w454) -> ("error out"=w453:errorcluster, "Goal 2"=w450:string, "File Path 2"=w449:path, "Experiment Name 2"=w451:string, "Add Entry Pressed?"=w452:bool)  [unwired: 6 in]
            n181 = case shown="True" w452 {
              tunnel: w451 -> [_ w460]
              tunnel: w450 -> [_ w459]
              tunnel: w449 -> [_ w458]
              frame False {
              }
              frame True {
                "Experiment Name" <- w460
                "Goal" <- w459
                "File Path" <- w458
              }
            }
          }
          event "Enable\nAutomatic\nRecording": Value Change {
            n182 = event-data() -> ("NewVal"=w461:bool)  [unwired: 1 in, 5 out]
            n183 = case shown="True" w461 {
              frame False {
              }
              frame True {
                n184 = property on="Stop" class="Bool (strict)"("Val(Sgnl)"=TRUE ("Value (Signaling)")) -> ()  [unwired: 2 in, 2 out]
              }
            }
          }
          event "Cycles": Value Change {
            n185 = event-data() -> ()  [unwired: 1 in, 6 out]
            n186 = call "Write Repeats.vi"("error in (no error)"=w475, "Repeats"="Cycles", "RampProgramModel in"=w476) -> ("error out"=w474:errorcluster, "RampProgramModel out"=w473:refnum<class "RampProgramModel.lvclass">)  [unwired: 7 in]
          }
          event "LoadProgram": Value Change {
            n187 = event-data() -> ()  [unwired: 1 in, 6 out]
            n188 = call-poly <vilib>:"Read From Spreadsheet File.vi"() -> ("all rows"=w480:dbl[][])  [unwired: 7 in, 4 out]
            n189 = call "WriteRampTable.vi"("RampFromFile"=w480, "RampProgramModel in"=w482) -> ("RampProgramModel out"=w481:refnum<class "RampProgramModel.lvclass">)  [unwired: 8 in, 1 out]
          }
          event "SaveProgram": Value Change {
            n190 = event-data() -> ()  [unwired: 1 in, 6 out]
            n191 = call "GetRampTable.vi"("error in (no error)"=w490, "RampProgramModel in"=w491) -> ("error out"=w488:errorcluster, "RampTable"=w487:string[][], "RampProgramModel out"=w489:refnum<class "RampProgramModel.lvclass">)  [unwired: 7 in]
            n192 = call-poly <vilib>:"Write To Spreadsheet File.vi"("2D data"=w487) -> ()  [unwired: 7 in, 1 out]
          }
          event "PauseProgram": Value Change {
            n193 = event-data() -> ()  [unwired: 1 in, 6 out]
          }
          event "RunProgram": Value Change {
            w503 = T4."Disabled and Grayed Out" ("Disabled")
            n194 = event-data() -> ()  [unwired: 1 in, 6 out]
            n195 = Not Equal?(x=w502, y=RampState."Pause Program" ("State")) -> (x != y?=w500:bool)
            n196 = property on="SaveProgram" class="Bool"("DisabledEnum"=w503) -> ()  [unwired: 2 in, 2 out]
            n197 = property on="LoadProgram" class="Bool"("DisabledEnum"=w503) -> ()  [unwired: 2 in, 2 out]
            n198 = property on="Clear Table" class="Bool"("DisabledEnum"=w503) -> ()  [unwired: 2 in, 2 out]
            n199 = property on="RunProgram" class="Bool"("DisabledEnum"=w503) -> ()  [unwired: 2 in, 2 out]
            n200 = case shown="True" w500 {
              frame False {
              }
              frame True {
                n201 = property on="Temp Chart" class="WFChart (strict)"("History Data"=dbl[] []) -> ()  [unwired: 2 in, 2 out]
              }
            }
          }
          event "StopProgram": Value Change {
            n202 = event-data() -> ()  [unwired: 1 in, 6 out]
          }
          event "Add Entry": Value Change {
            n203 = event-data() -> ()  [unwired: 1 in, 6 out]
            n204 = call "TableEntry.vi"("error in (no error)"=w525) -> ("error out"=w521:errorcluster, "Dwell Time @ SP (sec) 2"=w522:u32, "Cooling rate (°C/min) 2"=w523:dbl, "SP (°C) 2"=w524:dbl, "Add Entry Pressed?"=w526:bool)  [unwired: 6 in]
            n205 = case shown="True" w526 {
              tunnel: w524 -> [_ w535]
              tunnel: w523 -> [_ w534]
              tunnel: w522 -> [_ w533]
              tunnel: w521 -> [w528 w532]
              tunnel: [w528 w529] -> w520
              tunnel: w518 -> [w527 w531]
              tunnel: [w527 w530] -> w519
              frame False {
              }
              frame True {
                n206 = call "AddEntry2Table.vi"("Dwell Time @ SP (sec)"=w533, "error in (no error)"=w532, "Cooling rate (°C/min)"=w534, "SP (°C)"=w535, "RampProgramModel in"=w531) -> ("error out"=w529:errorcluster, "RampProgramModel out"=w530:refnum<class "RampProgramModel.lvclass">)  [unwired: 5 in]
              }
            }
          }
          event "Clear Table": Value Change {
            n207 = event-data() -> ()  [unwired: 1 in, 6 out]
            n208 = call "WriteRampTable.vi"("error in (no error)"=w542, "RampFromFile"=dbl[][] [], "RampProgramModel in"=w543) -> ("error out"=w541:errorcluster, "RampProgramModel out"=w540:refnum<class "RampProgramModel.lvclass">)  [unwired: 7 in]
          }
        }
        n209 = local read "stop"() -> (w246:bool)
        "Ramp Controller" <- w243
      }
    }
    frame Error {
    }
  }
  n210 = property class="IMAQdx"(reference=w7, "VideoMode"=u32 8) -> (reference out=w6:T3)  [unwired: 1 in, 1 out]
  n211 = call <vilib>:"IMAQdx Configure Grab.vi"("error in"=w47, "Session In"=w6) -> ("error out"=w46:errorcluster, "Session Out"=w10:T3)  [unwired: 8 out]
  n212 = call <vilib>:"IMAQdx Enumerate Attributes.vi"("Session In"=w10) -> ()  [unwired: 8 in, 3 out]
  n213 = call <vilib>:"IMAQdx Enumerate Video Modes.vi"("Session In"=w10) -> ()  [unwired: 7 in, 4 out]
  n214 = property class="IMAQdx" props=["BitsPerPixel", "VideoMode", "ActiveAttribute"](reference=w10) -> ()  [unwired: 1 in, 5 out]
  n215 = call "IMAQ Create"("Image Name"="Grab and Save to AVI Acq", "error in (no error)"=w46) -> ("New Image"=w45:T2, "error out"=w39:errorcluster)  [unwired: 2 in, 1 out]
  n216 = while {
    shift-right: [w553] -> _
    shift-left: AVI_recoder_state."Stop" -> [w558]
    tunnel: w29 -> [w557]
    tunnel: "error in (no error) 2" -> [w556]
    tunnel: [w555] -> w13
    shift-right: [w551] -> _
    shift-left: AVI_recoder_state."Stop" -> [w552]
    shift-right: [w550] -> _
    shift-left: T6 refnum ("AVI Refnum") -> [w549]
    shift-right: [w548] -> _
    shift-left: TRUE -> [w548]
    shift-right: [w546] -> _
    shift-left: w11 -> [w547]
    stop <- w559 continue-if-true
    n217 = event shown="[4] \"Stop\": Value Change" {
      selector: _ -> [_ _ _ _ _]
      dyn-events: _ -> [_ _ _ _ _]
      timeout: w557 -> [_ _ _ _ _]
      tunnel: w558 -> [w572 w647 w662 w678 _]
      tunnel: w556 -> [w571 w649 w654 w676 w689]
      tunnel: [w570 w643 w653 w676 w685] -> w555
      tunnel: [w569 _ _ _ _] -> w554
      tunnel: [w568 w647 w663 w679 AVI_recoder_state."Stop"] -> w553
      tunnel: w552 -> [w567 w646 _ _ w702]
      tunnel: [w566 w646 w662 w678 w702] -> w551
      tunnel: [w565 w648 w661 w677 w701] -> w550
      tunnel: w549 -> [w564 w648 w661 w677 w701]
      tunnel: w547 -> [w563 w634 w652 w675 w684]
      tunnel: [w562 w634 w652 w675 w684] -> w546
      event Timeout {
        n218 = event-data() -> ()  [unwired: 1 in, 3 out]
        n219 = case shown="\"Init\"" w572 {
          selector: w572 -> [w585 w590 w607 w632]
          tunnel: [w583 w592 w595 w628] -> w570
          tunnel: w571 -> [w575 w592 w609 w629]
          tunnel: [w583 w592 w596 w628] -> w569
          tunnel: [w585 w590 w607 AVI_recoder_state."Record"] -> w568
          tunnel: w567 -> [_ _ w606 _]
          tunnel: [w585 w590 w607 w632] -> w566
          tunnel: [w586 w591 T6 refnum ("AVI Refnum") w622] -> w565
          tunnel: w564 -> [w587 w591 w610 _]
          tunnel: w563 -> [w582 w588 w593 _]
          tunnel: [w581 w588 w593 w616] -> w562
          frame "Record", Default {
            (unwired) "%c" ("time format string (%c)")
            n220 = local read "Temp String (C)"() -> (w580:string)
            n221 = Format Date/Time String(time format string (%c)="%d/%%m/%Y %H:%M:%S%2u") -> (date/time string=w578:string)  [unwired: 2 in]
            n222 = call "Image-GFV.vi"("error in (no error)"=w575, "Image GFV Enum"=ImageEnum4GFV."Read") -> ("error out"=w574:errorcluster, "Output Image"=w573:T2)  [unwired: 8 in]
            n223 = Bundle("date/time string"=w578, "Temp String (C)"=w580) -> (w579:T12)  [unwired: 1 in]
            n224 = Build Array (concatenate)(w582, w579) -> (w581:T5)
            n225 = local write "Status"("Recording" ("Recorder Status")) -> ()
            n226 = call "IMAQ AVI2 Write Frame"("error in (no error)"=w574, "Image"=w573, "AVI Refnum"=w587) -> ("error out"=w583:errorcluster, "AVI Refnum (duplicate)"=w586:T6)  [unwired: 6 in, 1 out]
          }
          frame "Pause" {
            n227 = local write "Status"("Pause" ("Recorder Status")) -> ()
          }
          frame "Stop" {
            n228 = local read "Experiment Name"() -> (w603:string)
            n229 = Equal?(x=w607, y=w606) -> (x = y?=w605:bool)
            n230 = local read "File Path"() -> (w604:path)
            n231 = case shown="True" w605 {
              tunnel: w610 -> [w613 _]
              tunnel: w609 -> [w612 w614]
              tunnel: [w611 w614] -> w596
              frame False {
                n232 = call "IMAQ AVI2 Close"("error in (no error)"=w612, "AVI Refnum"=w613) -> ("error out"=w611:errorcluster)  [unwired: 9 in]
              }
              frame True {
              }
            }
            n233 = Empty String/Path?(string/path=w604) -> (empty?=w601:bool)
            n234 = Empty String/Path?(string/path=w603) -> (empty?=w602:bool)
            n235 = Or(x=w601, y=w602) -> (x .or. y?=w600:bool)
            n236 = Select(t=T4."Disabled and Grayed Out" ("Disabled"), s=w600, f=T4."Enabled" ("Disabled")) -> (s? t:f=w594:T4)
            n237 = property on="Record" class="Bool (strict)"(error in=w596, "DisabledEnum"=w594) -> (error out=w595:errorcluster)  [unwired: 1 in, 1 out]
            "Status" <- "Stop" ("Recorder Status")
          }
          frame "Init" {
            w616 = T5 []  # Date and Temp Cluster
            # "Create a file"
            n238 = call "IMAQ AVI2 Get Codec Names"() -> ("Codec Names"=w631:string[])  [unwired: 10 in, 1 out]
            n239 = local read "Experiment Name"() -> (w625:string)
            n240 = local read "File Path"() -> (w626:path)
            n241 = Index Array(array=w631, index="index 2") -> (element=w627:string)
            "Codec Type" <- w627
            n242 = Format Date/Time String(time format string (%c)="%d_%m_%Y-%H_%M_%S") -> (date/time string=w618:string)  [unwired: 2 in]
            n243 = Concatenate Strings(w625, "-" ("string"), w618, ".avi" ("string")) -> (w624:string)
            n244 = Build Path(base path=w626, name or relative path=w624) -> (appended path=w623:path)
            "Full avi Path and Name" <- w623
            n245 = call "IMAQ AVI2 Create"("error in (no error)"=w629, "Codec"=w627, "Frames Per Second"=u32 1, "AVI Path"=w623) -> ("error out"=w628:errorcluster, "AVI Refnum"=w622:T6)  [unwired: 6 in]
            n246 = local write "Status"("Init" ("Recorder Status")) -> ()
          }
        }
      }
      event "TakeRefImage": Value Change {
        n247 = event-data() -> ()  [unwired: 1 in, 6 out]
        n248 = call "Image-GFV.vi"("error in (no error)"=w649, "Image GFV Enum"=ImageEnum4GFV."Read") -> ("error out"=w644:errorcluster, "Output Image"=w645:T2)  [unwired: 8 in]
        "Reference Image" <- w645
        n249 = local read "Experiment Name"() -> (w641:string)
        n250 = local read "File Path"() -> (w642:path)
        n251 = Format Date/Time String(time format string (%c)="%d_%m_%Y-%H_%M_%S") -> (date/time string=w637:string)  [unwired: 2 in]
        n252 = Concatenate Strings(w641, "-" ("string"), w637, ".png" ("string")) -> (w640:string)
        n253 = Build Path(base path=w642, name or relative path=w640) -> (appended path=w636:path)
        n254 = call-poly "IMAQ Write File 2"("error in (no error)"=w644, "File Path"=w636, "Image"=w645) -> ("error out"=w643:errorcluster)  [unwired: 7 in, 1 out]
      }
      event "Record": Value Change {
        n255 = event-data() -> ()  [unwired: 1 in, 6 out]
        n256 = local read "Experiment Name"() -> (w659:string)
        n257 = local read "File Path"() -> (w660:path)
        n258 = local write "Record"(FALSE ("Record")) -> ()
        n259 = Empty String/Path?(string/path=w660) -> (empty?=w657:bool)
        n260 = Empty String/Path?(string/path=w659) -> (empty?=w658:bool)
        n261 = Or(x=w657, y=w658) -> (x .or. y?=w656:bool)
        n262 = Not(x=w656) -> (.not. x?=w655:bool)
        n263 = case shown="True" w655 {
          tunnel: [w665 w672] -> w663
          tunnel: w662 -> [w665 w671]
          tunnel: w654 -> [w664 w667]
          tunnel: [w664 w666] -> w653
          frame False {
          }
          frame True {
            n264 = property on="NewExperiment" class="Bool"(error in=w667, "DisabledEnum"=T4."Disabled and Grayed Out" ("Disabled")) -> (error out=w666:errorcluster)  [unwired: 1 in, 1 out]
            n265 = Equal?(x=w671, y=AVI_recoder_state."Stop") -> (x = y?=w669:bool)
            n266 = Select(t=AVI_recoder_state."Init", s=w669, f=AVI_recoder_state."Record") -> (s? t:f=w672:T7)
          }
        }
      }
      event "Pause": Value Change {
        n267 = event-data() -> ()  [unwired: 1 in, 6 out]
        n268 = Equal?(x=w678, y=AVI_recoder_state."Record") -> (x = y?=w681:bool)
        n269 = Select(t=AVI_recoder_state."Pause", s=w681, f=w678) -> (s? t:f=w679:T7)
      }
      event "Stop": Value Change {
        # "Save Ascii file with Experiments details"
        n270 = event-data() -> ()  [unwired: 1 in, 6 out]
        n271 = local read "Experiment Name"() -> (w690:string)
        n272 = local read "Goal"() -> (w691:string)
        n273 = local read "File Path"() -> (w694:path)
        n274 = local read "Ramp Program Table"() -> (w695:string[][])
        n275 = local read "Full avi Path and Name"() -> (w699:path)
        n276 = property on="Mag" class="Enum (strict)"() -> ("RingText.Text"=w698:string)  [unwired: 2 in, 2 out]
        n277 = local write "Stop"(FALSE ("Stop")) -> ()
        n278 = local read "Cycles"() -> (w697:u32)
        n279 = Path To String(path=w694) -> (string=w693:string)
        n280 = Number To Decimal String(number=w697) -> (decimal integer string=w696:string)  [unwired: 1 in]
        n281 = Bundle By Name(cluster=T11 {"Experiment Name"="", "Goal"="", "Remarks"="", "File Path"="", "Mag"="", "Repeat Program Number"="", "Full avi Path and Name"=path "", "Ramp Table "=[], "Date and Time"=[]} ("Ascii Experiment Data"), "Experiment Name"=w690, "Goal"=w691, "Remarks"="Remarks", "File Path"=w693, "Ramp Table"=w695, "Repeat Program Number"=w696, "Mag"=w698, "Full avi Path and Name"=w699, "Date and Time"=w684) -> (w688:T11)
        n282 = call "SaveExperimentDataToAsciiFile.vi"("error in (no error)"=w689, "Ascii Experiment Data"=w688) -> ("error out"=w686:errorcluster)  [unwired: 9 in]
        n283 = property on="NewExperiment" class="Bool"(error in=w686, "DisabledEnum"=T4."Enabled" ("Disabled")) -> (error out=w685:errorcluster)  [unwired: 1 in, 1 out]
      }
    }
    n284 = Unbundle By Name(w554) -> ("status"=w560:bool)
    n285 = local read "stop"() -> (w561:bool)
    n286 = Not Or(1:w561, 2:w560) -> (0:w559:bool)
    "Video Recorder" <- w548
  }
  n287 = call "Image-GFV.vi"("error in (no error)"=w39, "Image GFV Enum"=ImageEnum4GFV."Init") -> ("error out"=w38:errorcluster)  [unwired: 8 in, 1 out]
  n288 = while {
    tunnel: w10 -> [w750]
    tunnel: w38 -> [w749]
    tunnel: [w723] -> w42
    tunnel: [w722] -> w41
    shift-right: [w729] -> _
    shift-left: TRUE -> [w729]
    shift-right: ["High Resolution"] -> _
    shift-left: FALSE ("High Resolution") -> [w725]
    shift-right: [w720] -> w44
    shift-left: w45 -> [w719]
    shift-right: [w709] -> _
    shift-left: 0.0 ("Shutter (1-4095)") -> [w715]
    shift-right: [w710] -> _
    shift-left: 0.0 ("Gain (0-570)") -> [w714]
    stop <- w746 continue-if-true
    # "Changing Exposure and Gain"
    # "For Changing Resolution"
    n289 = local read "Experiment Name"() -> (w733:string)
    n290 = Wait (ms)(milliseconds to wait=u32 10) -> ()  [unwired: 1 out]
    n291 = local read "Status of Temperature Controller"() -> (w738:string)
    n292 = property on="Cooling Rate (°C/min)" class="DigNum (strict)"() -> ("Value"=w736:dbl)  [unwired: 2 in, 2 out]
    n293 = local read "Setpoint (°C)"() -> (w728:dbl)
    n294 = local read "Temp String (C)"() -> (w737:string)
    n295 = Number To Fractional String(number=w736, precision (6)=i16 2) -> (F-format string=w734:string)  [unwired: 2 in]
    n296 = Number To Fractional String(number=w728, precision (6)=i16 1) -> (F-format string=w727:string)  [unwired: 2 in]
    n297 = Bundle By Name(cluster=T13 {"Status"="", "Experiment Name"="", "Current Temp (C)"="", "Set Point (C)"="", "Cooling Rate (C/min)"="", "Mag"=enum."20x_LM"} ("TextOnImage"), "Current Temp (C)"=w737, "Set Point (C)"=w727, "Status"=w738, "Mag"="Mag", "Experiment Name"=w733, "Cooling Rate (C/min)"=w734) -> (w739:T13)
    n298 = call <vilib>:"IMAQdx Grab.vi"("error in"=w749, "Image In"=w719, "Session In"=w750) -> ("error out"=w742:errorcluster, "Image Out"=w743:T2, "Session Out"=w718:T3)  [unwired: 1 in, 5 out]
    n299 = call "AddText2Image.vi"("error in (no error)"=w742, "High Resolution"="High Resolution", "TextOnImage"=w739, "Input Image"=w743) -> ("error out"=w741:errorcluster, "Output Image"=w731:T2)  [unwired: 6 in]
    n300 = local read "Status"() -> (w732:string)
    n301 = Unbundle By Name(w741) -> ("status"=w748:bool)
    n302 = call "Image-GFV.vi"("error in (no error)"=w741, "Input Image"=w731, "Image GFV Enum"=ImageEnum4GFV."Write") -> ("error out"=w730:errorcluster)  [unwired: 7 in, 1 out]
    n303 = local read "stop"() -> (w747:bool)
    n304 = Not Or(1:w747, 2:w748) -> (0:w746:bool)
    n305 = call "AddRecordingOverlay2Image.vi"("error in (no error)"=w730, "Recording Status String"=w732, "Input Image"=w731) -> ("error out"=w707:errorcluster, "Output Image"=→"Image":T2)  [unwired: 7 in]
    n306 = Not Equal?(x=w715, y="Shutter (1-4095)") -> (x != y?=w717:bool)
    n307 = Not Equal?(x=w714, y="Gain (0-570)") -> (x != y?=w716:bool)
    n308 = Or(x=w717, y=w716) -> (x .or. y?=w713:bool)
    n309 = case shown="True" w713 {
      tunnel: w718 -> [w752 w759]
      tunnel: "Shutter (1-4095)" -> [_ w757]
      tunnel: "Gain (0-570)" -> [_ w756]
      tunnel: [w752 w755] -> w708
      tunnel: w707 -> [w751 w754]
      tunnel: [w751 w753] -> w706
      frame False {
      }
      frame True {
        n310 = property class="IMAQdx"(reference=w759, error in=w754, "ActiveAttribute"="CameraAttributes::Shutter::Value", "ValueDBL"=w757, "ActiveAttribute"="CameraAttributes::Gain::Value", "ValueDBL"=w756) -> (reference out=w755:T3, error out=w753:errorcluster)
      }
    }
    n311 = Not Equal?(x=w725, y="High Resolution") -> (x != y?=w724:bool)
    n312 = case shown="True" w724 {
      tunnel: w708 -> [w765 w788]
      tunnel: [w765 w779] -> w723
      tunnel: "High Resolution" -> [_ w778]
      tunnel: w706 -> [w763 w777]
      tunnel: [w763 w772] -> w722
      tunnel: w719 -> [w764 w775]
      tunnel: [w764 w767] -> w720
      tunnel: "Gain (0-570)" -> [w762 _]
      tunnel: "Shutter (1-4095)" -> [w761 _]
      tunnel: [w762 w766] -> w710
      tunnel: [w761 w766] -> w709
      frame False {
      }
      frame True {
        w766 = 0.0 ("Gain (0-570)")
        n313 = local read "Session In"() -> (w787:T3)
        n314 = call <vilib>:"IMAQdx Close Camera.vi"("error in"=w777, "Session In"=w788) -> ("error out"=w789:errorcluster)  [unwired: 9 out]
        n315 = call <vilib>:"IMAQdx Open Camera.vi"("error in"=w789, "Session In"=w787) -> ("error out"=w782:errorcluster, "Session Out"=w783:T3)  [unwired: 1 in, 7 out]
        n316 = Select(t=u32 15 ("f"), s=w778, f=u32 8) -> (s? t:f=w784:u32)
        n317 = property class="IMAQdx"(reference=w783, error in=w782, "VideoMode"=w784) -> (reference out=w781:T3, error out=w780:errorcluster)
        n318 = call <vilib>:"IMAQdx Configure Grab.vi"("error in"=w780, "Session In"=w781) -> ("error out"=w776:errorcluster, "Session Out"=w779:T3)  [unwired: 8 out]
        n319 = call "IMAQ Dispose"("Image"=w775, "error in (no error)"=w776) -> ("error out"=w770:errorcluster)  [unwired: 1 in, 3 out]
        n320 = call "Image-GFV.vi"("error in (no error)"=w770, "Image GFV Enum"=ImageEnum4GFV."Delete") -> ("error out"=w769:errorcluster)  [unwired: 8 in, 1 out]
        n321 = call "IMAQ Create"("Image Name"="New Grab", "error in (no error)"=w769) -> ("New Image"=w767:T2, "error out"=w773:errorcluster)  [unwired: 2 in, 1 out]
        n322 = call "Image-GFV.vi"("error in (no error)"=w773, "Image GFV Enum"=ImageEnum4GFV."Init") -> ("error out"=w772:errorcluster)  [unwired: 8 in, 1 out]
      }
    }
    "Video Grabber" <- w729
  }
  n323 = flat-sequence {
    tunnel: w17 -> [w790]
    tunnel: [w790] -> w16
    frame #0 {
      n324 = local write "Linkam Controller"(FALSE ("Linkam Controller")) -> ()
    }
  }
  n325 = flat-sequence {
    tunnel: w13 -> [w792]
    tunnel: [w792] -> w12
    frame #0 {
      n326 = local write "Video Recorder"(FALSE ("Video Recorder")) -> ()
    }
  }
  n327 = flat-sequence {
    tunnel: w19 -> [w794]
    tunnel: [w794] -> w18
    frame #0 {
      n328 = local write "Ramp Controller"(FALSE ("Ramp Controller")) -> ()
    }
  }
  n329 = VISA Close(VISA resource name=w55, error in (no error)=w16) -> (error out=w25:errorcluster)
  n330 = call <vilib>:"IMAQdx Close Camera.vi"("error in"=w41, "Session In"=w42) -> ("error out"=w43:errorcluster)  [unwired: 9 out]
  n331 = Merge Errors(w12, w14, w25, w18) -> (w24:errorcluster)
  n332 = call "IMAQ Dispose"("Image"=w44, "error in (no error)"=w43) -> ("error out"=w15:errorcluster)  [unwired: 1 in, 3 out]
  n333 = flat-sequence {
    tunnel: w24 -> [w796]
    tunnel: [w796] -> w23
    frame #0 {
      n334 = local write "stop"(FALSE ("stop")) -> ()
    }
  }
  n335 = flat-sequence {
    tunnel: w15 -> [w798]
    tunnel: [w798] -> w14
    frame #0 {
      n336 = local write "Video Grabber"(FALSE ("Video Grabber")) -> ()
    }
  }
  n337 = call "Image-GFV.vi"("error in (no error)"=w23, "Image GFV Enum"=ImageEnum4GFV."Delete") -> ("error out"=w37:errorcluster)  [unwired: 8 in, 1 out]
  n338 = call <vilib>:"Simple Error Handler.vi"("error in (no error)"=w37) -> ()  [unwired: 2 in, 7 out]
